vi "SetupSweepAndGetPeak.vi"(6 "Route Names":string[](array[string]), 7 "Cal?":bool, 8 "error in (no error)":errorcluster, 9 "Span(Hz)":dbl=26500000000.0, 10 "Center Frequency (Hz)":dbl=13250000000.0, 11 "Instrument in":refnum<class "Instrument.lvclass">) -> (0 "error out":errorcluster, 1 "FDelta(hz)":dbl, 2 "Calibrated Amplitude (dBm)":dbl, 3 "Instrument out":refnum<class "Instrument.lvclass">)   [LabVIEW 2014, in "Instrument.lvclass"]
uses:
  Instrument.lvclass
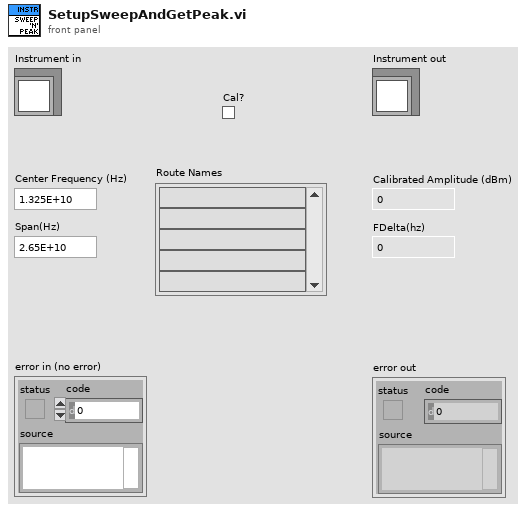
[diagram p1: front panel]
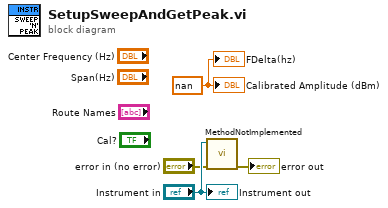
[diagram p0: block diagram]
diagram:
  w4 = nan ("Calibrated Amplitude (dBm)")
  n1 = call "MethodNotImplemented.vi"("error in (no error)"="error in (no error)", "LabVIEW Object In"="Instrument in") -> ("error out"=→"error out":errorcluster)  [unwired: 9 in]
  "Instrument out" <- "Instrument in"
  "FDelta(hz)" <- w4
  "Calibrated Amplitude (dBm)" <- w4
